vi "TCP Engine JSON to LabVIEW Data.vi"(8 "error in":errorcluster, 11 "JSON String":string) -> (0 "error out":errorcluster, 1 "SubCmd":string, 2 "Command":string, 3 "Interface":string, 5 "Data":variant)   [LabVIEW 2018, in "TCP Engine.lvlib"]
doc: "All Rights Reserved © 2017 SyncSols"
uses:
  TCP Engine.lvlib
  <vilib>/Utility/error.llb/Error Cluster From Error Code.vi
  <vilib>/ErrorRing/Error Ring.xnode
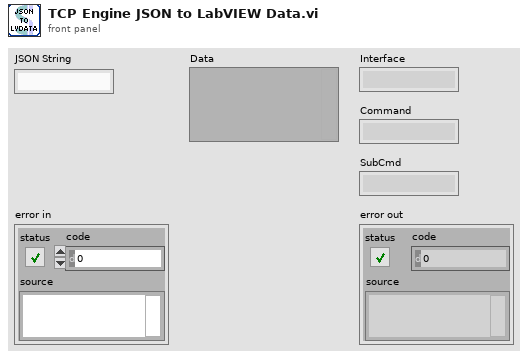
[diagram p1: front panel]
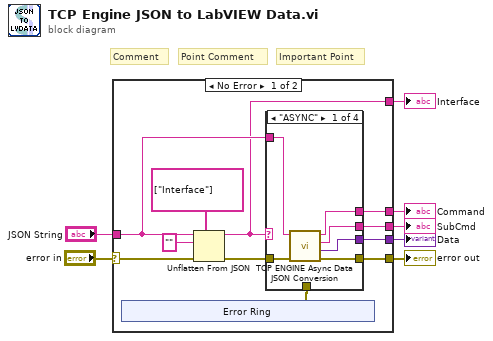
[diagram p0: block diagram]
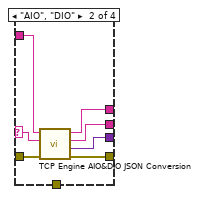
[diagram p2: hidden frame]
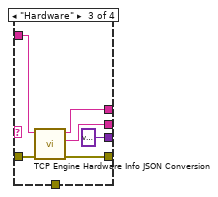
[diagram p3: hidden frame]
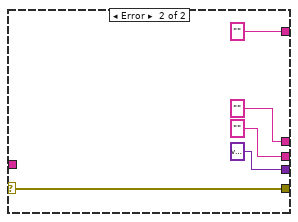
[diagram p5: hidden frame]
diagram:
  # "Important Point"
  # "Point Comment"
  # "Comment"
  n1 = case shown="No Error" "error in" {
    selector: "error in" -> [w18 w48]
    tunnel: [w13 w48] -> w7
    tunnel: "JSON String" -> [w14 _]
    tunnel: [w12 variant ("Data")] -> w2
    tunnel: [w11 "" ("SubCmd")] -> w3
    tunnel: [w10 "" ("Command")] -> w4
    tunnel: [w9 ""] -> w1
    frame No Error {
      n2 = xnode "Error Ring"() -> ("error out"=w8:errorcluster)
      n3 = Unflatten From JSON(path=string[] ["Interface"], JSON string=w14, type and defaults="", error in (no error)=w18) -> (value=w9:string, error out=w15:errorcluster)  [unwired: 3 in]
      n4 = case shown="\"ASYNC\"" w9 {
        selector: w9 -> [_ w30 _ _]
        tunnel: w15 -> [w29 w36 w42 _]
        tunnel: w14 -> [w28 w35 w37 _]
        tunnel: [w27 w34 w41 w43] -> w13
        tunnel: [w26 w33 w40 _] -> w10
        tunnel: [w25 w32 w39 _] -> w11
        tunnel: [w24 w31 variant ("Data") _] -> w12
        tunnel: w8 -> [_ _ _ w43]
        frame "ASYNC" {
          n5 = call "TCP ENGINE Async Data JSON Conversion.vi"("error in"=w29, "JSON String"=w28) -> ("error out"=w27:errorcluster, "Data"=w24:variant, "SubCmd"=w25:string, "Command"=w26:string)  [unwired: 6 in]
        }
        frame "AIO", "DIO" {
          n6 = call "TCP Engine AIO&DIO JSON Conversion.vi"("error in"=w36, "Interface"=w30, "JSON String"=w35) -> ("error out"=w34:errorcluster, "Data"=w31:variant, "SubCmd"=w32:string, "Command"=w33:string)  [unwired: 5 in]
        }
        frame "Hardware" {
          n7 = call "TCP Engine Hardware Info JSON Conversion.vi"("error in"=w42, "JSON String"=w37) -> ("error out"=w41:errorcluster, "Sub Command"=w39:string, "Command"=w40:string)  [unwired: 7 in]
        }
        frame Default {
        }
      }
    }
    frame Error {
    }
  }
  "error out" <- w7
  "Command" <- w4
  "SubCmd" <- w3
  "Data" <- w2
  "Interface" <- w1
